vi "动态调用.vi"(8 "错误输入":errorcluster, 11 "VI路径":path) -> (0 "错误输出":errorcluster)   [LabVIEW 2014]
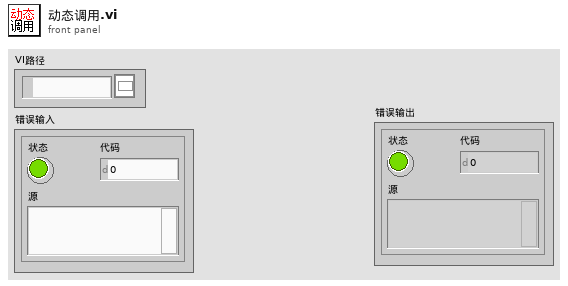
[diagram p1: front panel]
types:
  T1 = enum32{"Invalid", "Standard", "Closed", "Hidden", "Minimized", "Maximized"}
  T2 = enum32{"Bad", "Idle", "Run top level", "Running"}
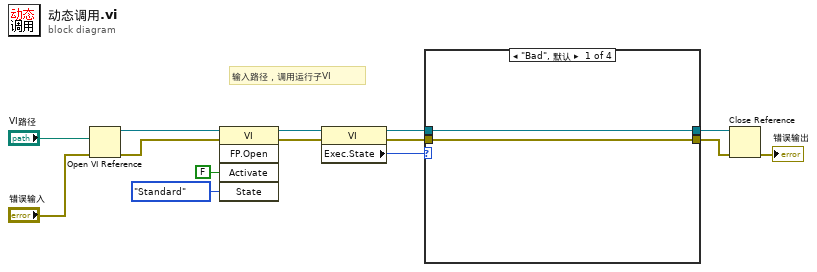
[diagram p0: block diagram]
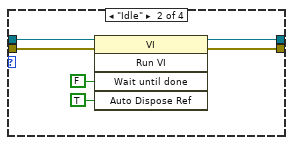
[diagram p2: hidden frame]
diagram:
  # "输入路径，调用运行子VI"
  n1 = Open VI Reference(vi path="VI路径", error in (no error)="错误输入") -> (vi reference=w12:refnum<vi>, error out=w11:errorcluster)  [unwired: 4 in]
  n2 = invoke class="VI" method="FP.Open"(reference=w12, error in=w11, "Activate"=FALSE ("激活？"), "State"=T1."Standard" ("状态")) -> (reference out=w8:refnum<vi>, error out=w7:errorcluster)  [unwired: 1 in, 3 out]
  n3 = property class="VI"(reference=w8, error in=w7) -> (reference out=w5:refnum<vi>, error out=w4:errorcluster, "Exec.State"=w6:T2)
  n4 = case shown="\"Bad\", 默认" w6 {
    tunnel: w5 -> [w16 w22 w24 w26]
    tunnel: w4 -> [w15 w21 w23 w25]
    tunnel: [w16 w20 w24 w26] -> w3
    tunnel: [w15 w19 w23 w25] -> w2
    frame "Bad", Default {
    }
    frame "Idle" {
      n5 = invoke class="VI" method="Run VI"(reference=w22, error in=w21, "Wait until done"=FALSE ("结束前等待"), "Auto Dispose Ref"=TRUE ("自动销毁引用")) -> (reference out=w20:refnum<vi>, error out=w19:errorcluster)  [unwired: 1 in, 3 out]
    }
    frame "Run top level" {
    }
    frame "Running" {
    }
  }
  n6 = Close Reference(reference=w3, error in (no error)=w2) -> (error out=→"错误输出":errorcluster)
